vi "Select Correlation pairs.vi"(2 "Correlate In":i32[][](array[numeric]), 3 "Instrument names":string[](array[string])) -> (0 "Correlate Out":i32[][](array[numeric]))   [LabVIEW 2022 SP3]
panel:
  in  "OK":bool
  in  "Number of Pairs":i32
  in  "Pairs to Correlate":u16[][](array[ring]) items=["RV (P0)", "RV (P1)"]
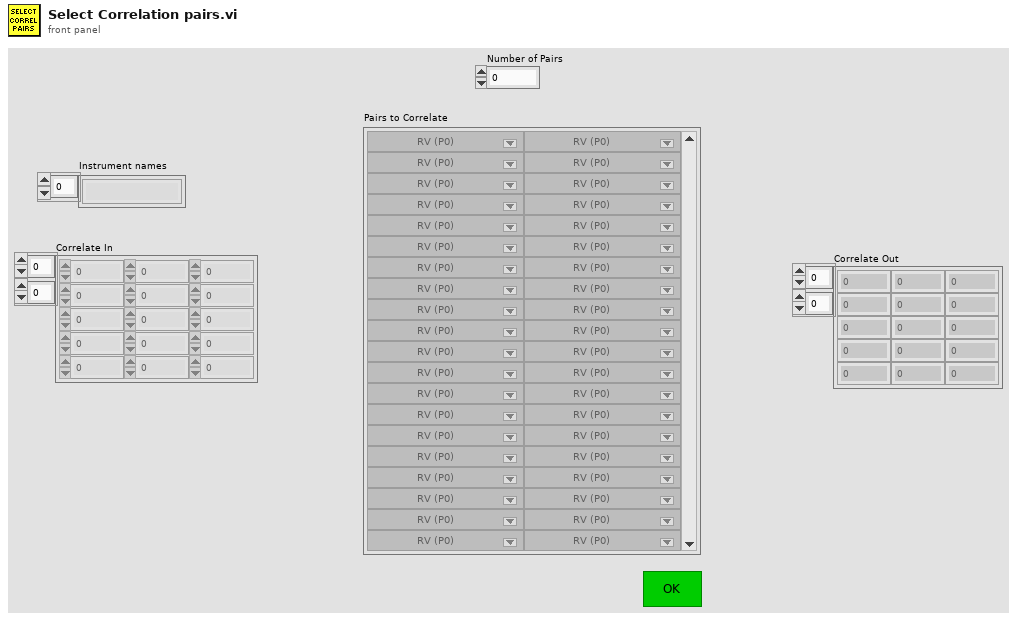
[diagram p1: front panel]
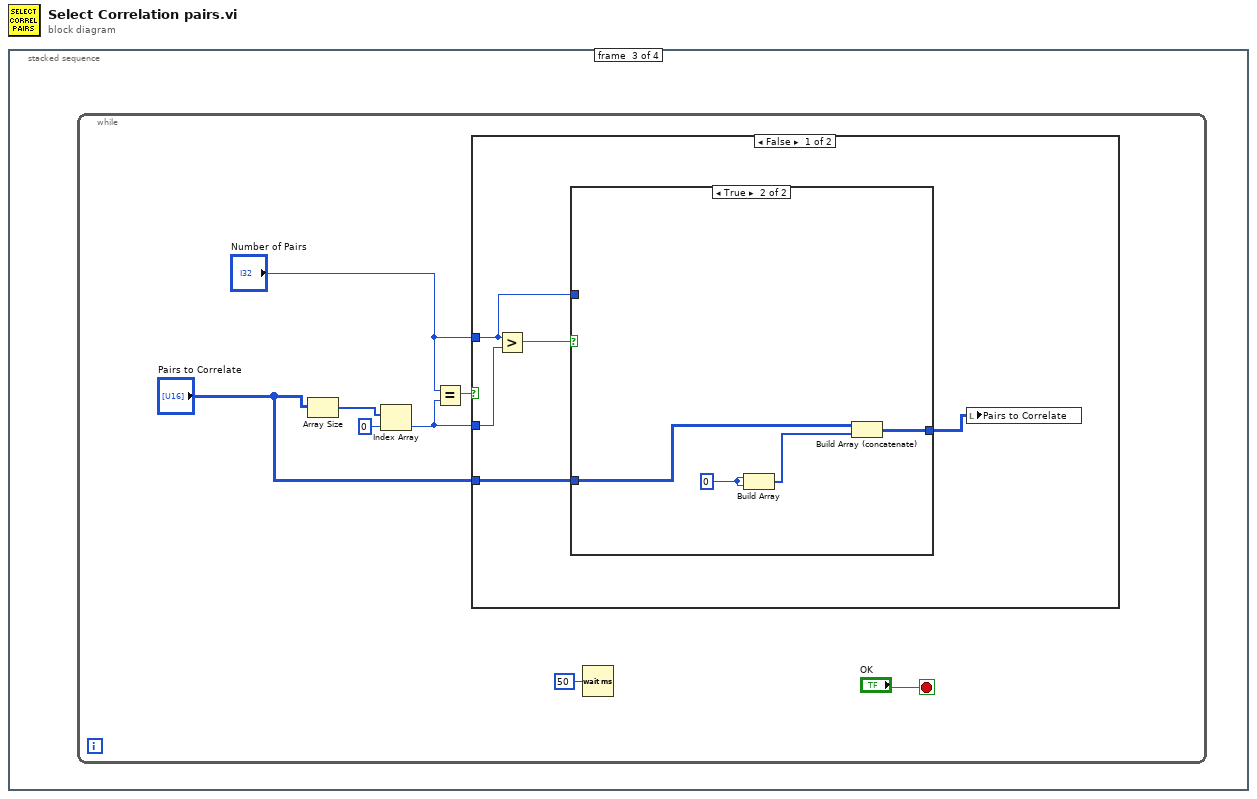
[diagram p0: block diagram]
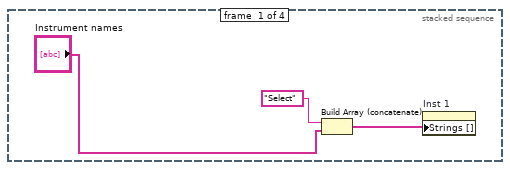
[diagram p2: hidden frame]
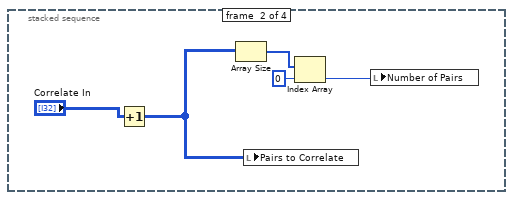
[diagram p3: hidden frame]
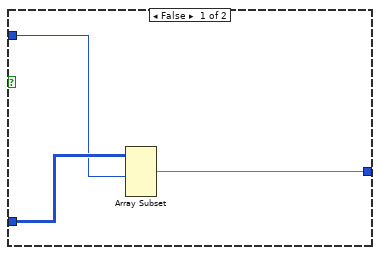
[diagram p4: hidden frame]
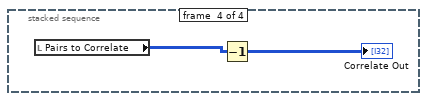
[diagram p6: hidden frame]
diagram:
  n1 = stacked-sequence {
    frame #0 {
      n2 = Build Array (concatenate)("Select", "Instrument names") -> (w1:string[])
      n3 = property on="Inst 1" class="Ring (strict)"("Strings []"=w1) -> ()  [unwired: 2 in, 2 out]
    }
    frame #1 {
      n4 = Increment(x="Correlate In") -> (x+1=w4:i32[][])
      n5 = Array Size(array=w4) -> (size(s)=w8:i32[])
      n6 = local write "Pairs to Correlate"(w4) -> ()
      n7 = Index Array(array=w8, index=0) -> (element=w7:i32)
      n8 = local write "Number of Pairs"(w7) -> ()
    }
    frame #2 {
      n9 = while {
        stop <- "OK" stop-if-true
        n10 = Array Size(array="Pairs to Correlate") -> (size(s)=w16:i32[])
        n11 = Index Array(array=w16, index=0) -> (element=w11:i32)
        n12 = Equal?(x="Number of Pairs", y=w11) -> (x = y?=w14:bool)
        n13 = case shown="False" w14 {
          tunnel: "Number of Pairs" -> [w18 _]
          tunnel: "Pairs to Correlate" -> [w20 _]
          tunnel: w11 -> [w17 _]
          frame False {
            n14 = Greater?(x=w18, y=w17) -> (0:w21:bool)
            n15 = case shown="True" w21 {
              tunnel: w20 -> [w24 w28]
              tunnel: [w23 w27] -> w19
              tunnel: w18 -> [w22 _]
              frame False {
                n16 = Array Subset(array=w24, length (row)=w22) -> (w23:u16[][])  [unwired: 3 in]
              }
              frame True {
                w25 = 0 ("Inst 1")
                n17 = Build Array(w25, w25) -> (w26:i32[])
                n18 = Build Array (concatenate)(w28, w26) -> (w27:i32[][])
              }
            }
            n19 = local write "Pairs to Correlate"(w19) -> ()
          }
          frame True {
          }
        }
        n20 = Wait (ms)(milliseconds to wait=u32 50) -> ()  [unwired: 1 out]
      }
    }
    frame #3 {
      n21 = local read "Pairs to Correlate"() -> (w30:u16[][])
      n22 = Decrement(x=w30) -> (x-1=→"Correlate Out":u16[][])
    }
  }
